vi "MODSWP MSMT Set Step Name.vi"(8 "error in (no error)":errorcluster, 10 "Step In":refnum<k7>, 11 "ModSweep in":refnum<class "ModSweep.lvclass">) -> (0 "error out":errorcluster, 2 "Step Out":refnum<k7>, 3 "ModSweep out":refnum<class "ModSweep.lvclass">)   [LabVIEW 2018, in "ModSweep.lvlib" / "ModSweep.lvclass"]
uses:
  ModSweep.lvclass
  Plugins/TestStand API Tools (TSAT).lvlibp/Step Actions/TSAT Step Actions.lvlib
  Plugins/String Database.lvlibp/String Database.lvclass
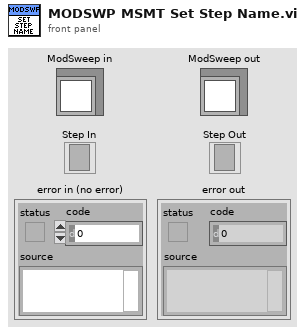
[diagram p1: front panel]
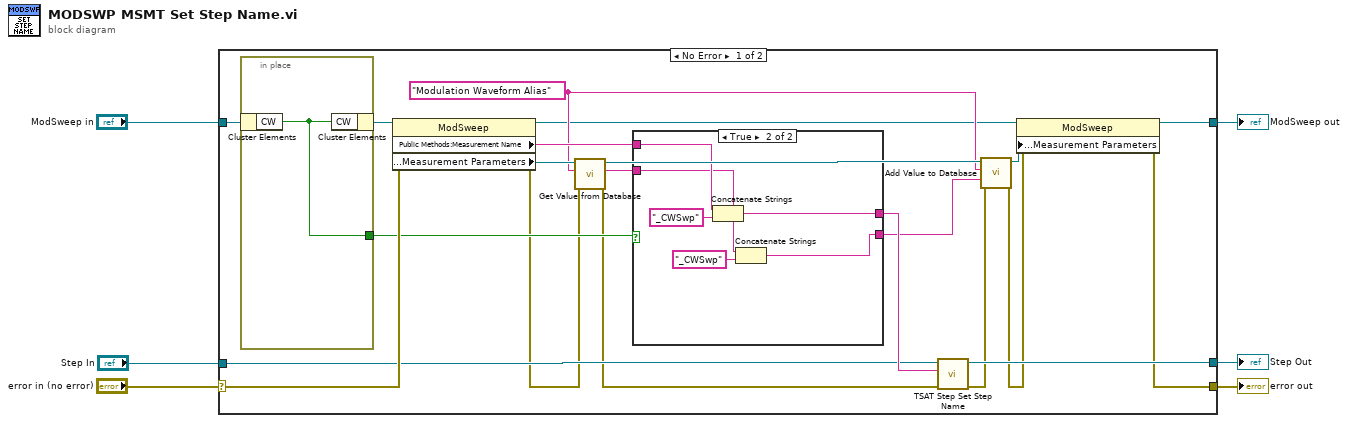
[diagram p0: block diagram]
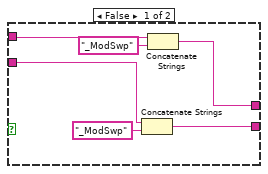
[diagram p2: hidden frame]
diagram:
  n1 = case shown="No Error" "error in (no error)" {
    selector: "error in (no error)" -> [w27 w43]
    tunnel: [w11 w43] -> w5
    tunnel: [w9 w42] -> w3
    tunnel: "ModSweep in" -> [w26 w42]
    tunnel: "Step In" -> [w21 w41]
    tunnel: [w20 w41] -> w1
    frame No Error {
      w15 = "Modulation Waveform Alias" ("Entry Name")
      n2 = in-place {
        in-place-border: [w40] -> w23
        n3 = in-place-cluster #1(w26) -> ("CW"=w40:bool)
        n4 = in-place-cluster #1("CW"=w40) -> (w25:refnum<class "ModSweep.lvclass">)
      }
      n5 = property class="ModSweep"(reference=w25, error in=w27) -> (reference out=w10:refnum<class "ModSweep.lvclass">, error out=w13:errorcluster, "Public Methods:Measurement Name"=w24:string, "Protected Methods:Measurement Parameters"=w19:refnum<class "String Database.lvclass">)
      n6 = call "Get Value from Database.vi"("error in (no error)"=w13, "Entry Name"=w15, "Message in"=w19) -> ("error out"=w12:errorcluster, "Entry Value"=w14:string, "Message out"=w18:refnum<class "String Database.lvclass">)  [unwired: 5 in, 1 out]
      n7 = case shown="True" w23 {
        tunnel: w24 -> [w32 w39]
        tunnel: [w33 w37] -> w22
        tunnel: w14 -> [w29 w35]
        tunnel: [w28 w34] -> w7
        frame False {
          n8 = Concatenate Strings(w29, "_ModSwp" ("string")) -> (w28:string)
          n9 = Concatenate Strings(w32, "_ModSwp" ("string")) -> (w33:string)
        }
        frame True {
          n10 = Concatenate Strings(w39, "_CWSwp" ("string")) -> (w37:string)
          n11 = Concatenate Strings(w35, "_CWSwp" ("string")) -> (w34:string)
        }
      }
      n12 = call "TSAT Step Set Step Name.vi"("Error In"=w12, "Name"=w22, "Step In"=w21) -> ("Error Out"=w17:errorcluster, "Step Out"=w20:refnum<k7>)  [unwired: 7 in]
      n13 = call "Add Value to Database.vi"("error in (no error)"=w17, "Entry Value"=w7, "Entry Name"=w15, "Dictionary In"=w18) -> ("error out"=w16:errorcluster, "Dictionary Out"=w8:refnum<class "String Database.lvclass">)  [unwired: 5 in, 1 out]
      n14 = property class="ModSweep"(reference=w10, error in=w16, "Protected Methods:Measurement Parameters"=w8) -> (reference out=w9:refnum<class "ModSweep.lvclass">, error out=w11:errorcluster)
    }
    frame Error {
    }
  }
  "error out" <- w5
  "ModSweep out" <- w3
  "Step Out" <- w1
